vi "Abort.vi"(8 "error in (no error)":errorcluster, 10 "Batch Group Number  (0: OFF)":i32(ring) items=["OFF", "1", "2", "3", "4", "5", "6", "7", "8", "9", "10", "11", "12", "ALL"], 11 "VISA resource name":refnum<visa-resource-name>) -> (0 "error out":errorcluster, 3 "VISA resource name out":refnum<visa-resource-name>)   [LabVIEW 2020, in "Yokogawa GX Series.lvlib"]
doc: "Aborts an acquisition and returns the oscilloscope to the Idle state. You initiate an acquisition with the <B>Initiate VI</B>.\n\n<B>Note</B> This VI does not check the instrument status. Typically, you call this VI only in a sequence of calls to other low-level instrument driver VIs. The sequence performs one operation. You use the low-level VIs to optimize one or more aspects of interaction with the instrument."
uses:
  <instrlib>/Yokogawa GX Series/Yokogawa GX Series.lvlib
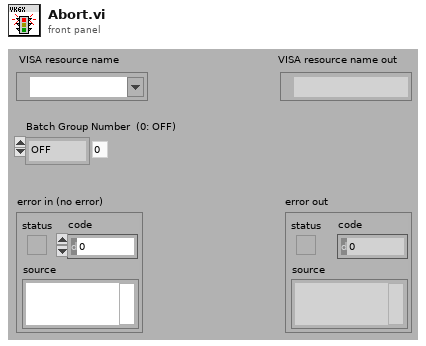
[diagram p1: front panel]
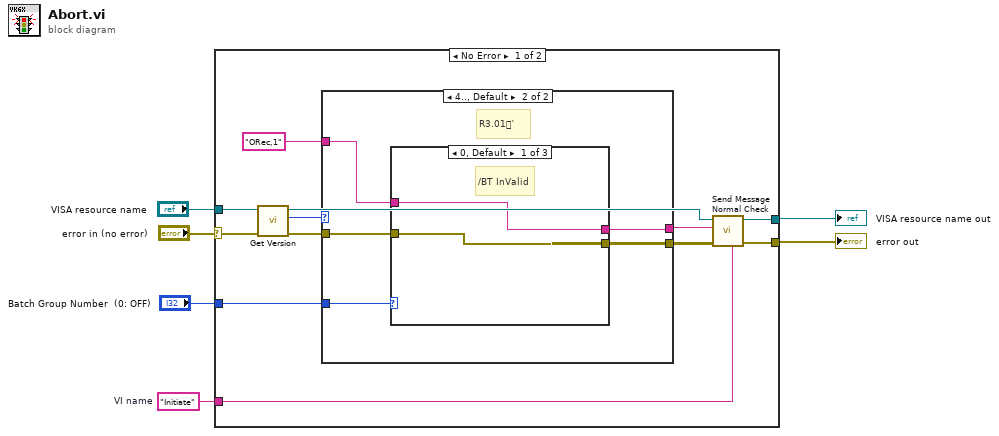
[diagram p0: block diagram]
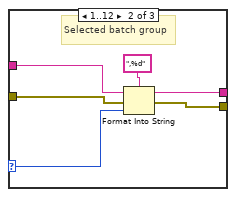
[diagram p3: hidden frame]
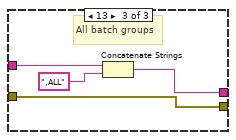
[diagram p4: hidden frame]
diagram:
  w4 = "Initiate"  # VI name
  n1 = case shown="No Error" "error in (no error)" {
    selector: "error in (no error)" -> [w14 w38]
    tunnel: "VISA resource name" -> [w15 w39]
    tunnel: [w18 w39] -> w6
    tunnel: [w17 w38] -> w5
    tunnel: w4 -> [w16 _]
    tunnel: "Batch Group Number  (0: OFF)" -> [w7 _]
    frame No Error {
      n2 = call <instrlib>:"Get Version.vi"("error in (no error)"=w14, "VISA resource name"=w15) -> ("error out"=w11:errorcluster, "Version"=w13:i32, "VISA resource name out"=w8:refnum<visa-resource-name>)  [unwired: 7 in]
      n3 = case shown="4.., Default" w13 {
        tunnel: "ORec,1" -> [w20 w24]
        tunnel: [w20 w21] -> w9
        tunnel: w11 -> [w19 w22]
        tunnel: [w19 w23] -> w10
        tunnel: w7 -> [_ w25]
        frame 0..3 {
          # "R1.03AR2.02AR2.03"
        }
        frame 4.., Default {
          # "R3.01`"
          n4 = case shown="0, Default" w25 {
            selector: w25 -> [_ w30 _]
            tunnel: [w26 w32 w34] -> w23
            tunnel: [w27 w31 w37] -> w21
            tunnel: w24 -> [w27 w29 w35]
            tunnel: w22 -> [w26 w28 w34]
            frame 0, Default {
              # "/BT InValid"
            }
            frame 1..12 {
              # "Selected batch group"
              n5 = Format Into String(format string=",%d", initial string=w29, error in=w28, w30) -> (resulting string=w31:string, error out=w32:errorcluster)
            }
            frame 13 {
              # "All batch groups"
              n6 = Concatenate Strings(w35, ",ALL") -> (w37:string)
            }
          }
        }
      }
      n7 = call <instrlib>:"Send Message Normal Check.vi"("Source (\"\")"=w16, "error in (no error)"=w10, "Send Message (\"\")"=w9, "VISA resource name"=w8) -> ("error out"=w17:errorcluster, "VISA resource name out"=w18:refnum<visa-resource-name>)  [unwired: 2 in, 4 out]
    }
    frame Error {
    }
  }
  "error out" <- w5
  "VISA resource name out" <- w6
